vi "case.vi"() -> ()   [LabVIEW 2016]
panel:
  in  "String":string
  out "Numeric Indicator":dbl
  in  "A 2":dbl
  in  "A":dbl
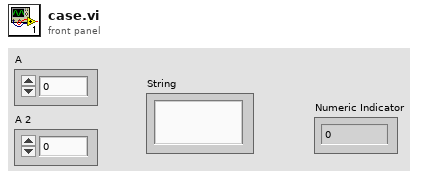
[diagram p1: front panel]
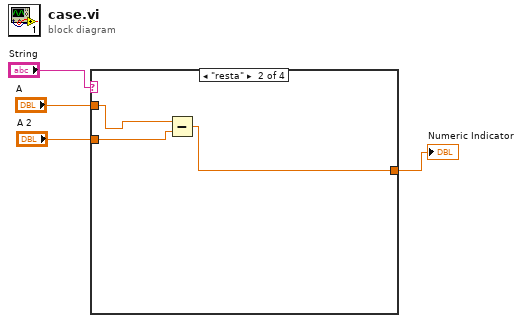
[diagram p0: block diagram]
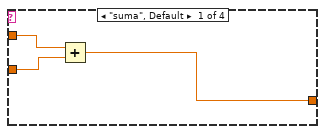
[diagram p2: hidden frame]
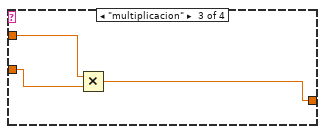
[diagram p3: hidden frame]
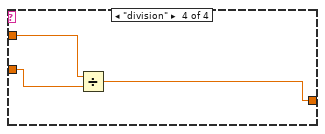
[diagram p4: hidden frame]
diagram:
  n1 = case shown="\"resta\"" "String" {
    tunnel: "A" -> [w7 w10 w12 w15]
    tunnel: "A 2" -> [w6 w9 w11 w14]
    tunnel: [w5 w8 w13 w16] -> w2
    frame "suma", Default {
      n2 = Add(x=w7, y=w6) -> (x+y=w5:dbl)
    }
    frame "resta" {
      n3 = Subtract(x=w10, y=w9) -> (x-y=w8:dbl)
    }
    frame "multiplicacion" {
      n4 = Multiply(x=w12, y=w11) -> (x*y=w13:dbl)
    }
    frame "division" {
      n5 = Divide(x=w15, y=w14) -> (x/y=w16:dbl)
    }
  }
  "Numeric Indicator" <- w2
